vi "StartTestSuite.vi"(8 "error in (no error)":errorcluster, 10 "TestSuite":refnum<class "TestSuite.lvclass">, 11 "EventTestListener in":refnum<class "EventTestListener.lvclass">) -> (0 "error out":errorcluster, 3 "EventTestListener out":refnum<class "EventTestListener.lvclass">)   [LabVIEW 2019, in "TestExplorer.lvlib" / "EventTestListener.lvclass"]
doc: "A test suite started."
uses:
  EventTestListener.lvclass
  TestSuite/TestSuite.lvclass
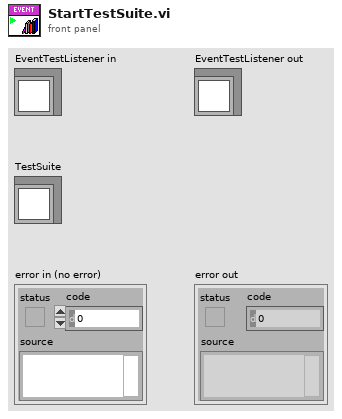
[diagram p1: front panel]
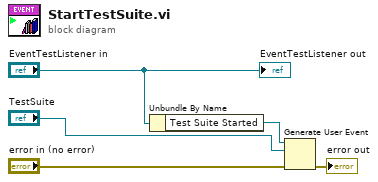
[diagram p0: block diagram]
diagram:
  n1 = Unbundle By Name("EventTestListener in") -> ("Test Suite Started"=w3:refnum<user-event>)
  n2 = Generate User Event(user event=w3, event data cluster="TestSuite", error in="error in (no error)") -> (error out=→"error out":errorcluster)  [unwired: 1 in, 1 out]
  "EventTestListener out" <- "EventTestListener in"
